vi "Config File Write.vi"(6 "Controls Excluded":refnum<vi>[](array[refnum]), 8 "Error In":errorcluster, 10 "Path":path, 11 "Controls In":refnum<vi>[](array[refnum])) -> (0 "Error Out":errorcluster, 2 "Path_Out":path)   [LabVIEW 2015]
uses:
  <vilib>/Utility/config.llb/Write Key (String).vi
  <vilib>/Utility/config.llb/NI_LVConfig.lvlib
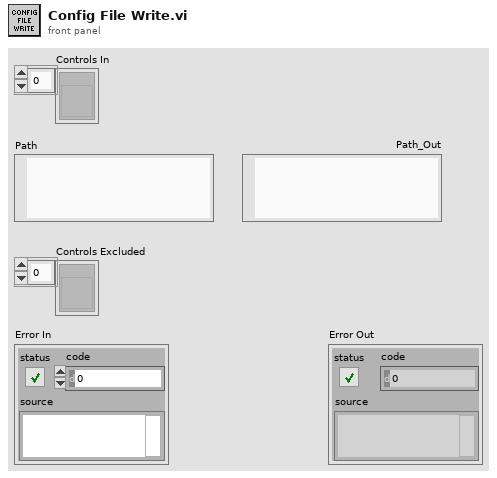
[diagram p1: front panel]
types:
  T1 = typedef "NI_LVConfig.lvlib/Config Data RefNum.ctl" = refnum<k1>
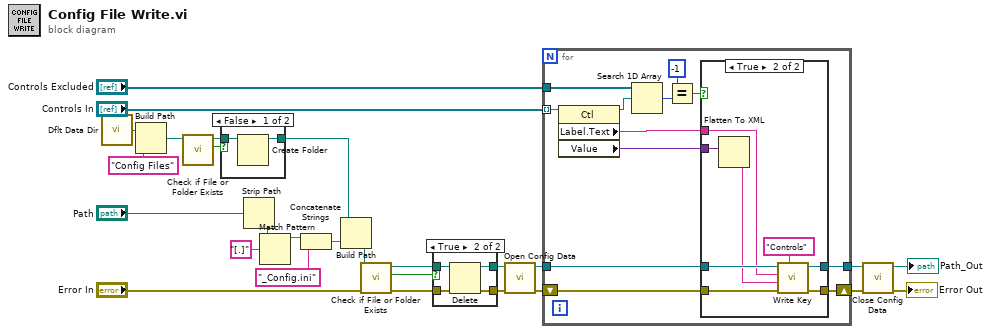
[diagram p0: block diagram]
diagram:
  n1 = call <vilib>:"Dflt Data Dir.vi"() -> ("App:Default Data Directory"=w7:path)
  n2 = Build Path(base path=w7, name or relative path="Config Files") -> (appended path=w5:path)
  n3 = call <vilib>:"Check if File or Folder Exists.vi"("path"=w5) -> ("file or folder exists?"=w3:bool, "dup path"=w4:path)  [unwired: 8 in, 1 out]
  n4 = case shown="False" w3 {
    tunnel: w4 -> [w29 w30]
    tunnel: [w28 w30] -> w2
    frame False {
      n5 = Create Folder(path (use dialog)=w29) -> (created path=w28:path)  [unwired: 2 in, 2 out]
    }
    frame True {
    }
  }
  n6 = Strip Path(path="Path") -> (name=w27:string)  [unwired: 1 out]
  n7 = Match Pattern(string=w27, regular expression="[.]" ("search string")) -> (before substring=w25:string)  [unwired: 1 in, 3 out]
  n8 = Concatenate Strings(w25, "_Config.ini") -> (w23:string)
  n9 = Build Path(base path=w2, name or relative path=w23) -> (appended path=w18:path)
  n10 = call <vilib>:"Check if File or Folder Exists.vi"("error in (no error)"="Error In", "path"=w18) -> ("error out"=w11:errorcluster, "file or folder exists?"=w12:bool, "dup path"=w10:path)  [unwired: 7 in]
  n11 = case shown="True" w12 {
    tunnel: w11 -> [w31 w36]
    tunnel: w10 -> [w32 w35]
    tunnel: [w32 w34] -> w9
    tunnel: [w31 w33] -> w8
    frame False {
    }
    frame True {
      n12 = Delete(path (use dialog)=w35, error in=w36) -> (deleted path=w34:path, error out=w33:errorcluster)  [unwired: 3 in, 1 out]
    }
  }
  n13 = call <vilib>:"Open Config Data.vi"("error in (no error)"=w8, "configuration file path"=w9) -> ("error out"=w15:errorcluster, "refnum"=w16:T1)  [unwired: 1 in, 7 out]
  n14 = for {
    shift-right: [w46] -> w14
    shift-left: w15 -> [w47]
    tunnel: "Controls In" -> [w43] mode=indexing
    tunnel: "Controls Excluded" -> [w41]
    tunnel: w16 -> [w48]
    tunnel: [w45] -> w13
    n15 = property class="Ctl"(reference=w43) -> (reference out=w42:refnum<vi>, "Label.Text"=w44:string, "Value"=w37:variant)  [unwired: 1 in, 1 out]
    n16 = Search 1D Array(1D array=w41, element=w42) -> (index of element=w40:i32)  [unwired: 1 in]
    n17 = Equal?(x=-1, y=w40) -> (x = y?=w38:bool)
    n18 = case shown="True" w38 {
      tunnel: w48 -> [w50 w58]
      tunnel: w47 -> [w49 w57]
      tunnel: [w49 w55] -> w46
      tunnel: [w50 w54] -> w45
      tunnel: w44 -> [_ w53]
      tunnel: w37 -> [_ w51]
      frame False {
      }
      frame True {
        n19 = Flatten To XML(anything=w51) -> (xml string=w52:string)
        n20 = call-poly <vilib>:"Write Key.vi"("section"="Controls", "error in (no error)"=w57, "value"=w52, "key"=w53, "refnum"=w58) -> ("error out"=w55:errorcluster, "refnum out"=w54:T1)  [unwired: 4 in, 1 out]
      }
    }
  }
  n21 = call <vilib>:"Close Config Data.vi"("error in (no error)"=w14, "refnum"=w13) -> ("error out"=→"Error Out":errorcluster, "file path"=→"Path_Out":path)  [unwired: 1 in, 7 out]
